vi "Enable Control.vi"(9 "enable":bool=TRUE, 11 "Control":refnum<vi>) -> ()   [LabVIEW 2018]
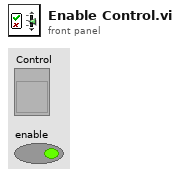
[diagram p1: front panel]
types:
  T1 = enum8{"Enabled", "Disabled", "Disabled and Grayed Out"}
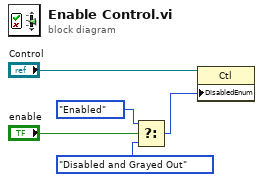
[diagram p0: block diagram]
diagram:
  n1 = Select(t=T1."Enabled" ("Disabled"), s="enable", f=T1."Disabled and Grayed Out" ("Disabled")) -> (s? t:f=w1:T1)
  n2 = property on="Property Node" class="Ctl"(reference="Control", "DisabledEnum"=w1) -> ()  [unwired: 1 in, 2 out]
